vi "add one color to Multi Listbox.vi"(6 "F： Clear Table Data":bool, 7 "ColumnNum":i32, 8 "error in (no error)":errorcluster, 9 "Row Num":i32=50, 10 "Color Box":u32(colorbox)=16448250, 11 "Multicolumn Listbox In":refnum<vi>) -> (0 "error out":errorcluster, 3 "Multicolumn Listbox Out":refnum<vi>)   [LabVIEW 2021]
uses:
  <vilib>/Utility/miscctls.llb/LVRowAndColumnTypeDef.ctl
  <vilib>/Utility/miscctls.llb/LVRowAndColumnUnsignedTypeDef.ctl
panel:
  in  "Color Box 2":u32(colorbox)=16448250
  out "size(s)":i32[](array[numeric])
  in  "Multicolumn Listbox":i32[](listbox)
  in  "s":bool
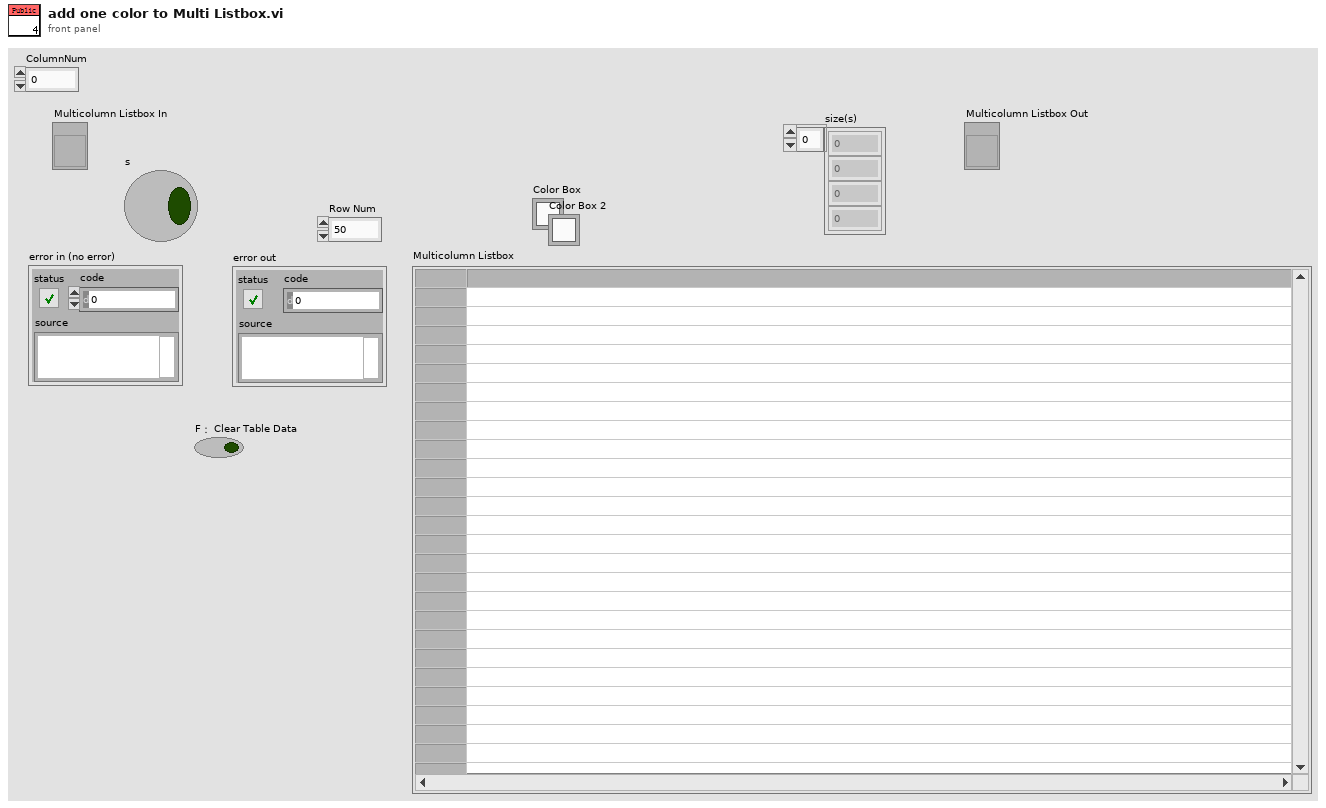
[diagram p1: front panel]
types:
  T1 = typedef "LVRowAndColumnTypeDef.ctl" = cluster{"Row":i32, "Column":i32}
  T2 = typedef "LVRowAndColumnUnsignedTypeDef.ctl" = cluster{"Row":u32, "Column":u32}
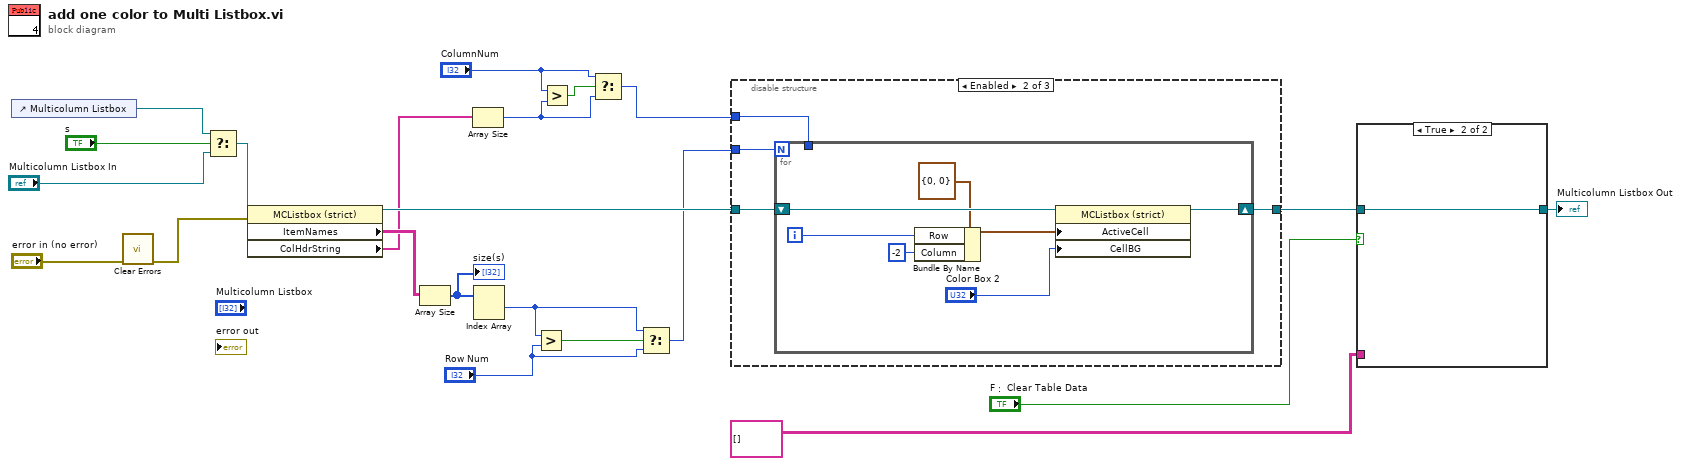
[diagram p0: block diagram]
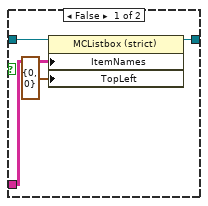
[diagram p2: hidden frame]
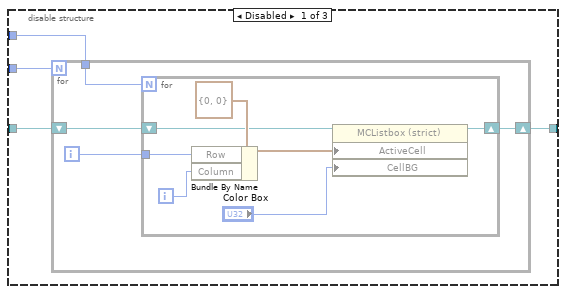
[diagram p3: hidden frame]
diagram:
  n1 = control-ref of="Multicolumn Listbox"() -> (w18:refnum<vi>)
  n2 = call <vilib>:"Clear Errors.vi"("error in (no error)"="error in (no error)") -> ("error out"=w17:errorcluster)  [unwired: 5 in, 1 out]
  n3 = Select(t=w18, s="s", f="Multicolumn Listbox In") -> (s? t:f=w20:refnum<vi>)
  n4 = property class="MCListbox (strict)"(reference=w20, error in=w17) -> (reference out=w15:refnum<vi>, "ItemNames"=w21:string[][], "ColHdrString"=w14:string[])  [unwired: 1 out]
  n5 = Array Size(array=w21) -> (size(s)=w22:i32[])
  "size(s)" <- w22
  n6 = Array Size(array=w14) -> (size(s)=w5:i32)
  n7 = Index Array(array=w22) -> (element #1=w9:i32)  [unwired: 2 in, 1 out]
  n8 = Greater?(x=w9, y="Row Num") -> (0:w11:bool)
  n9 = Greater?(x="ColumnNum", y=w5) -> (0:w7:bool)
  n10 = Select(t="ColumnNum", s=w7, f=w5) -> (s? t:f=w4:i32)
  n11 = Select(t=w9, s=w11, f="Row Num") -> (s? t:f=w8:i32)
  n12 = disable-structure shown="Enabled" {
    disable-tunnel: w15 -> [w26 w41 _]
    disable-tunnel: [w25 w40 _] -> w13
    disable-tunnel: w8 -> [w24 w39 _]
    disable-tunnel: w4 -> [w23 w38 _]
    frame Disabled {
      n13 = for {
        N: w24 -> [_]
        tunnel: w23 -> [w29]
        shift-right: [w27] -> w25
        shift-left: w26 -> [w28]
        i -> [w30]
        n14 = for {
          N: w29 -> [_]
          tunnel: w30 -> [w34]
          shift-right: [w32] -> w27
          shift-left: w28 -> [w33]
          i -> [w35]
          n15 = Bundle By Name(cluster=T1 {"Row"=0, "Column"=0} ("Active Cell:Active Cell"), "Row"=w34, "Column"=w35) -> (w36:T1)
          n16 = property on="Property Node" class="MCListbox (strict)"(reference=w33, "ActiveCell"=w36, "CellBG"="Color Box") -> (reference out=w32:refnum<vi>)  [unwired: 1 in, 1 out]
        }
      }
    }
    frame Enabled {
      n17 = for {
        N: w39 -> [_]
        tunnel: w38 -> [_]
        shift-right: [w46] -> w40
        shift-left: w41 -> [w47]
        i -> [w48]
        n18 = Bundle By Name(cluster=T1 {"Row"=0, "Column"=0} ("Active Cell:Active Cell"), "Row"=w48, "Column"=-2) -> (w44:T1)
        n19 = property on="Property Node" class="MCListbox (strict)"(reference=w47, "ActiveCell"=w44, "CellBG"="Color Box 2") -> (reference out=w46:refnum<vi>)  [unwired: 1 in, 1 out]
      }
    }
    frame Disabled {
    }
  }
  n20 = case shown="True" "F： Clear Table Data" {
    tunnel: w13 -> [w52 w53]
    tunnel: [w51 w53] -> w1
    tunnel: string[][] [] ("Item Names") -> [w50 _]
    frame False {
      n21 = property class="MCListbox (strict)"(reference=w52, "ItemNames"=w50, "TopLeft"=T2 {"Row"=0, "Column"=0} ("Top Left Visible Cell")) -> (reference out=w51:refnum<vi>)  [unwired: 1 in, 1 out]
    }
    frame True {
    }
  }
  "Multicolumn Listbox Out" <- w1
